vi "mqttCmdDatagram.vi"(8 "error in (no error)":errorcluster, 10 "byte1":u8, 11 "mqttBrokerCommand in":refnum<class "mqttCmd.lvclass">) -> (0 "error out":errorcluster, 2 "datagram":u8[](array[numeric]), 3 "mqttBrokerCommand out":refnum<class "mqttCmd.lvclass">)   [LabVIEW 2020, in "mqttCmd.lvclass"]
uses:
  mqttCmd.lvclass
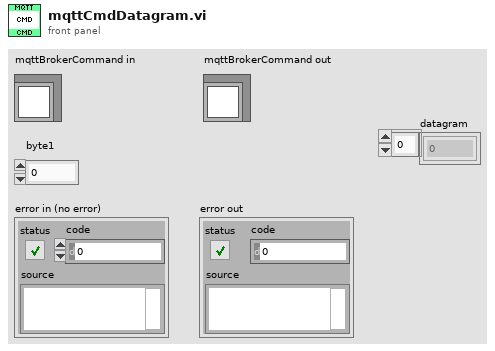
[diagram p1: front panel]
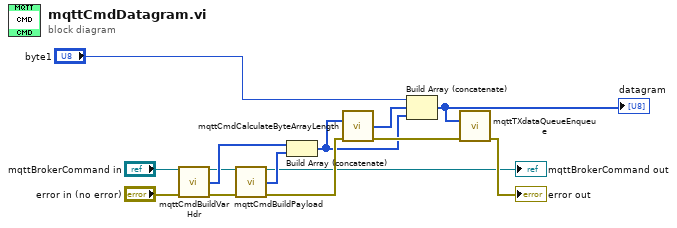
[diagram p0: block diagram]
diagram:
  n1 = call-dynamic "mqttCmdBuildVarHdr.vi"("_mqtt in"="mqttBrokerCommand in", "error in (no error)"="error in (no error)") -> ("_mqtt out"=w2:refnum<class "mqttCmd.lvclass">, "variableHeader"=w9:u8[], "error out"=w3:errorcluster)  [unwired: 11 in]
  n2 = call-dynamic "mqttCmdBuildPayload.vi"("_mqtt in"=w2, "error in (no error)"=w3) -> ("_mqtt out"=→"mqttBrokerCommand out":refnum<class "mqttCmd.lvclass">, "payload"=w10:u8[], "error out"=w8:errorcluster)  [unwired: 11 in]
  n3 = Build Array (concatenate)(w9, w10) -> (w7:u8[])
  n4 = call "mqttCmdCalculateByteArrayLength.vi"("byteArry in"=w7, "error in (no error)"=w8) -> ("length out"=w6:u8[], "error out"=w11:errorcluster)  [unwired: 12 in]
  n5 = Build Array (concatenate)("byte1", w6, w7) -> (w12:u8[])
  "datagram" <- w12
  n6 = call "mqttTXdataQueueEnqueue.vi"("data in"=w12, "error in (no error)"=w11) -> ("error out"=→"error out":errorcluster)  [unwired: 13 in]
